vi "Main VI.vi"(0 "Available Test":string(tree), 1 "Status and graph":bool, 5 "Home":bool, 7 "Mode selection":bool, 9 "Configuration":bool, 11 "Error In":errorcluster, 12 "Run Test":bool) -> (4 "Status":string, 15 "Error Out":errorcluster)   [LabVIEW 2020, in "ADC DAC Test Measurement.lvlib"]
doc: "Main interface VI to perform the tests. It performs INL and DNL Test. It contains individual button to load its corresponding page."
uses:
  ADC DAC Test Measurement.lvlib
  Typedef/Queue Operation.ctl
  Typedef/Data Line.ctl
  Class/Test/Parent/Test.lvclass
  Typedef/User event controls.ctl
  <vilib>/Utility/config.llb/Read Key (Boolean).vi
  <vilib>/Utility/config.llb/NI_LVConfig.lvlib
panel:
  out "Graph Pic":picture
  out "Config Pic":picture
  out "Mode Pic":picture
  out "Home Pic":picture
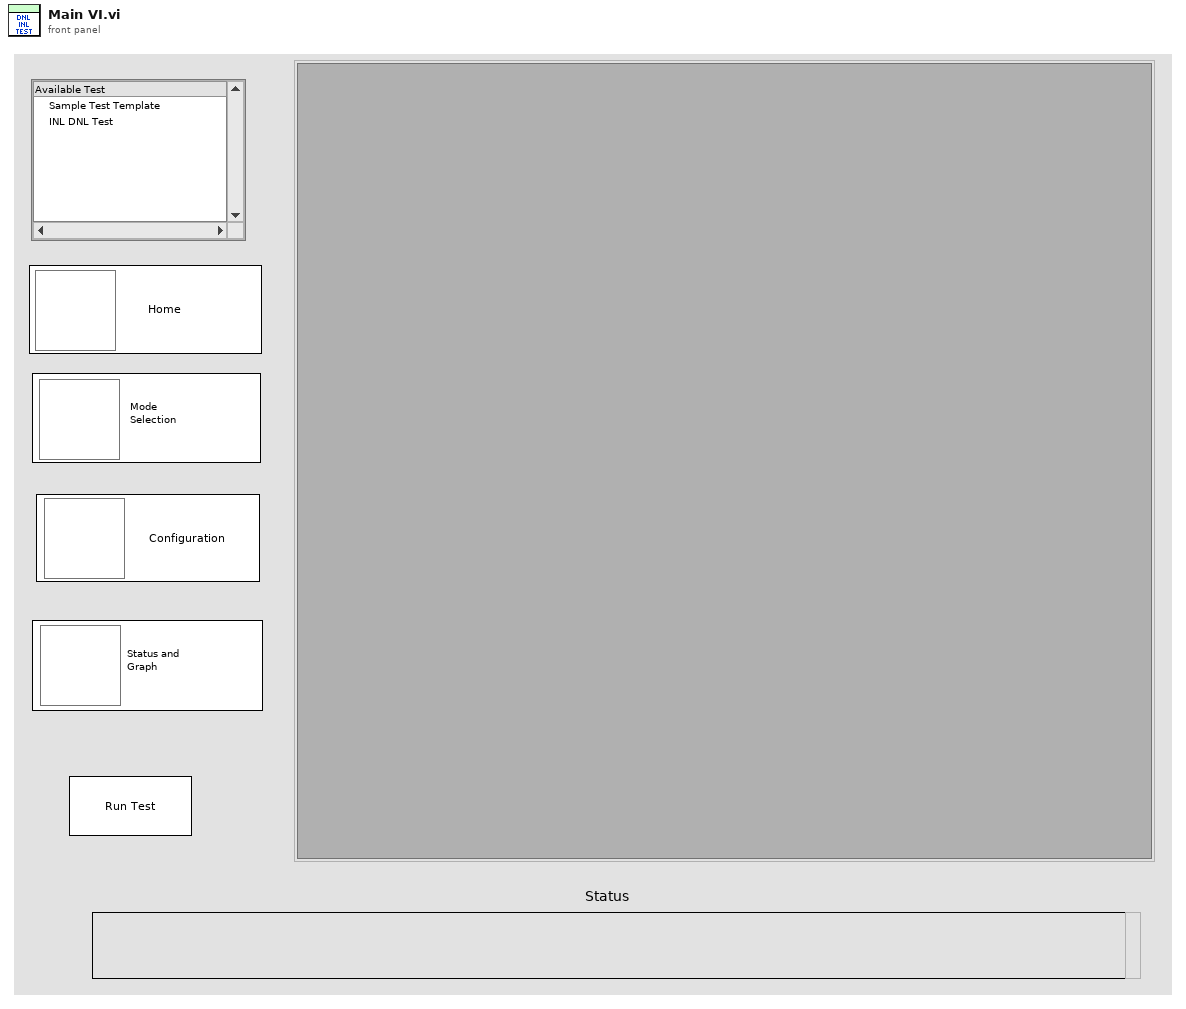
[diagram p1: front panel]
types:
  T1 = typedef "ADC DAC Test Measurement.lvlib/Data Line.ctl" = cluster{"DVR":refnum<data-value>, "Subpanel Ref":refnum<vi>, "Class Selected?":bool, "Status Msg":string, "Test Name":string, "Debug Status":bool}
  T2 = typedef "ADC DAC Test Measurement.lvlib/Queue Operation.ctl" = enum16{"Create Queue", "Enqueue", "Dequeue", "Enstack", "Flush Queue", "Release Queue"}
  T3 = typedef "ADC DAC Test Measurement.lvlib/User event controls.ctl" = enum16{"Create", "Generate", "Run Test", "Get Ref", "Destroy"}
  T4 = typedef "NI_LVConfig.lvlib/Config Data RefNum.ctl" = refnum<k1>
  T5 = typedef "imagedata.ctl" = cluster{"image type":i32, "image depth":i32, "image":u8[], "mask":u8[], "colors":u32[], "Rectangle":cluster{"left":i16, "top":i16, "right":i16, "bottom":i16}}
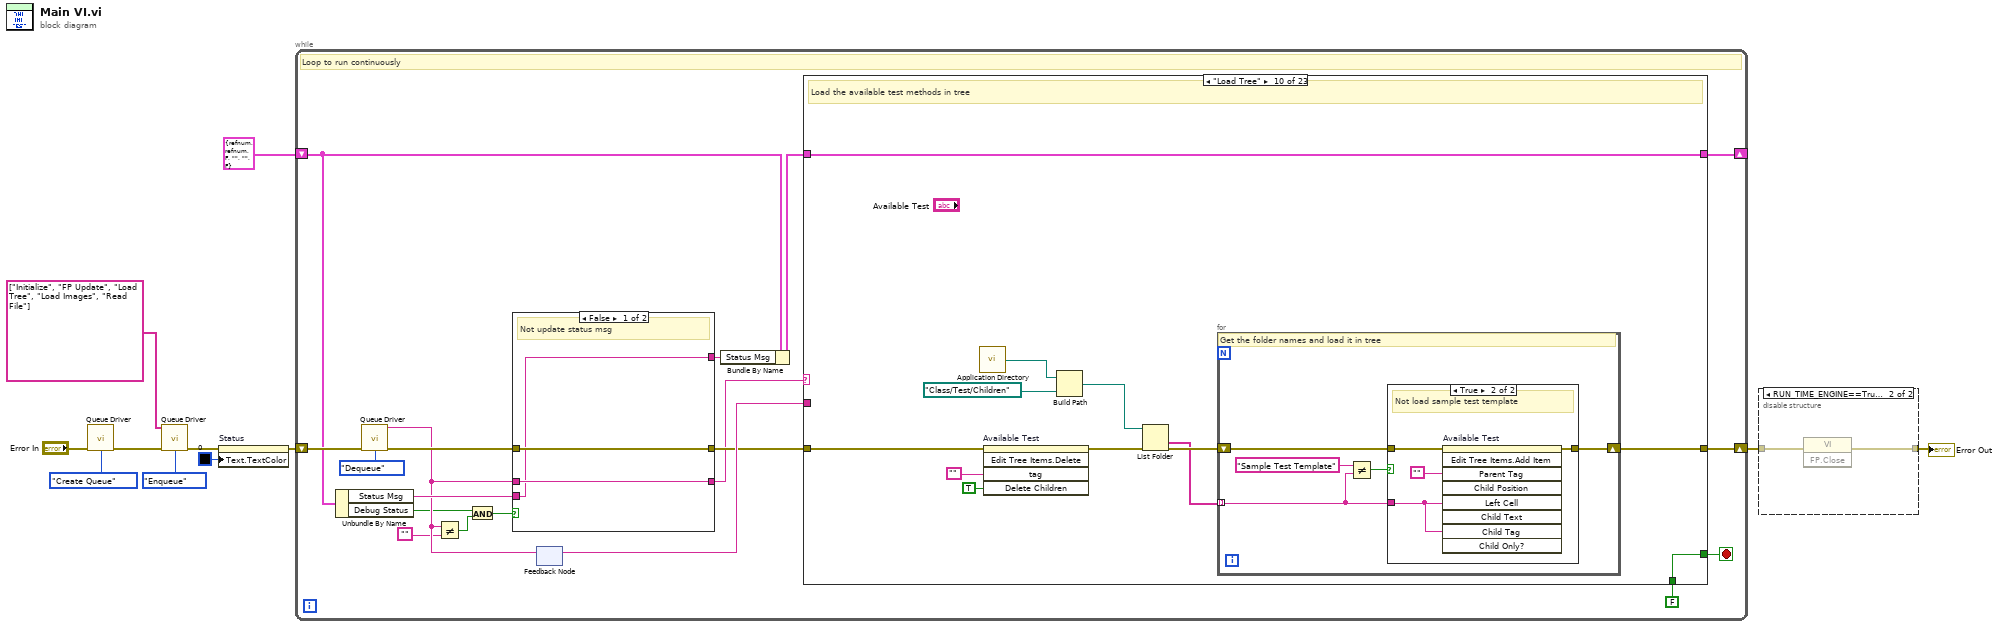
[diagram p0: block diagram]
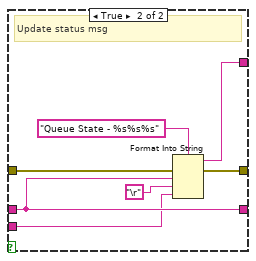
[diagram p3: hidden frame]
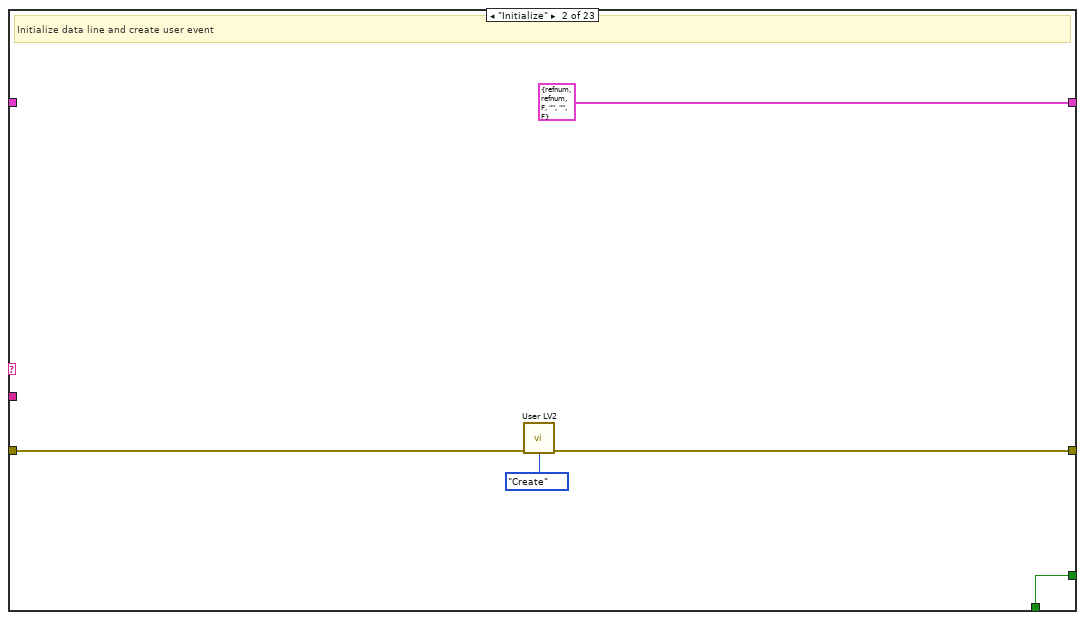
[diagram p5: hidden frame]
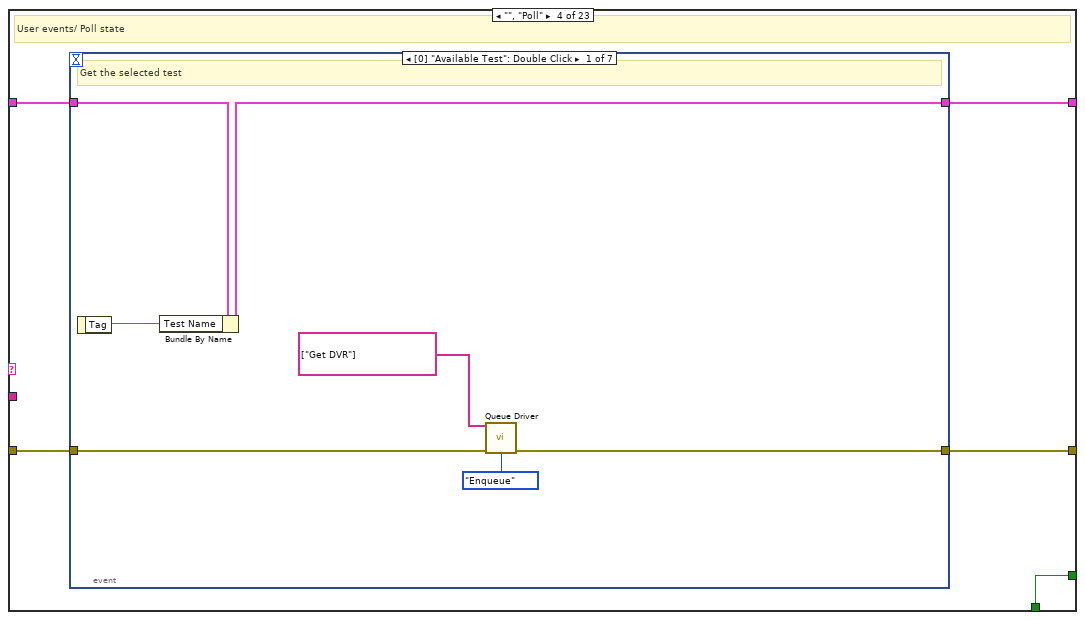
[diagram p7: hidden frame]
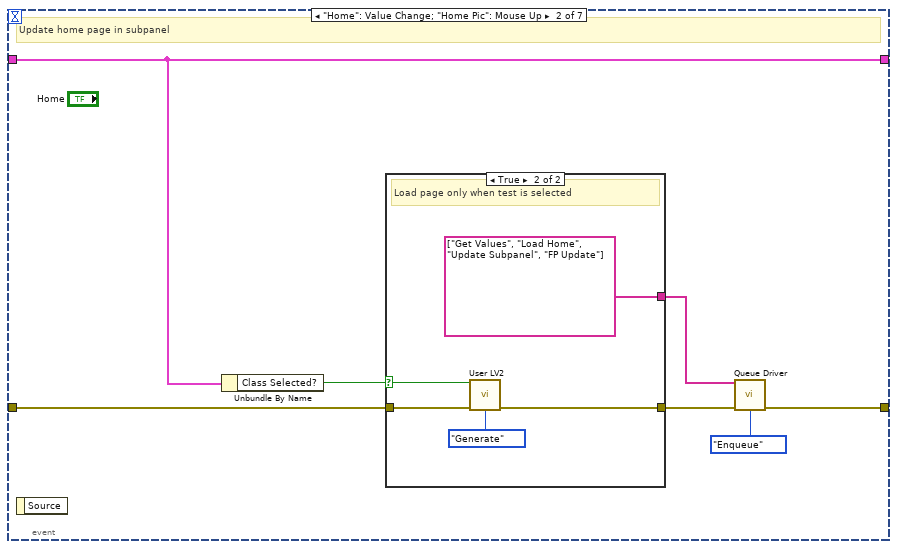
[diagram p8: hidden frame]
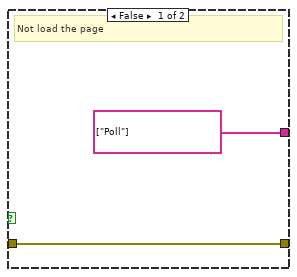
[diagram p9: hidden frame]
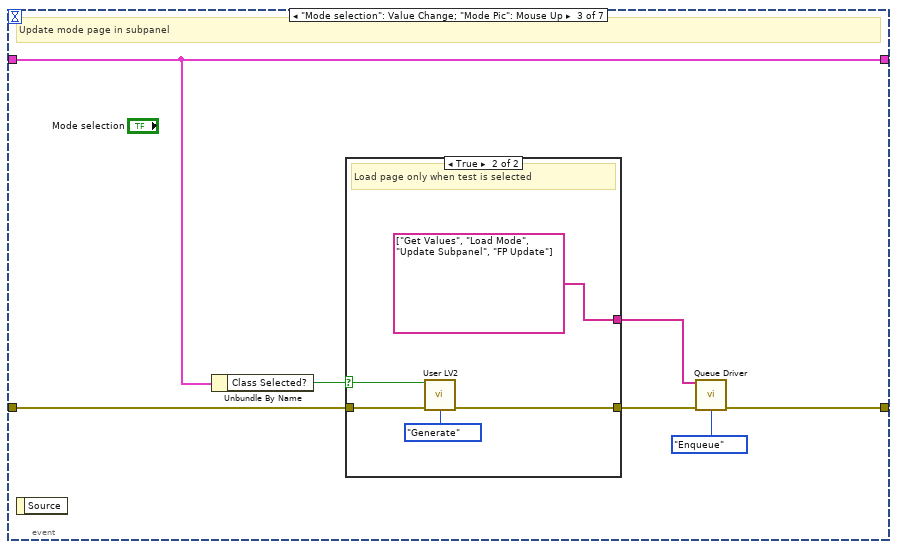
[diagram p10: hidden frame]
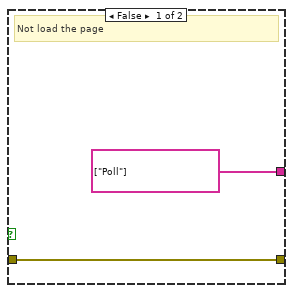
[diagram p11: hidden frame]
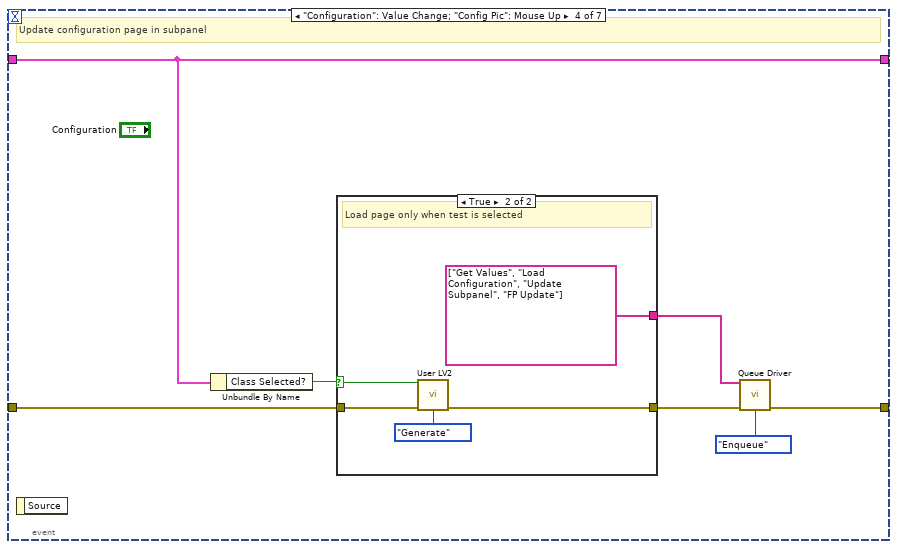
[diagram p12: hidden frame]
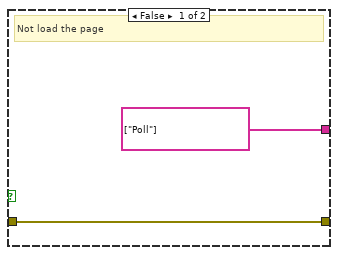
[diagram p13: hidden frame]
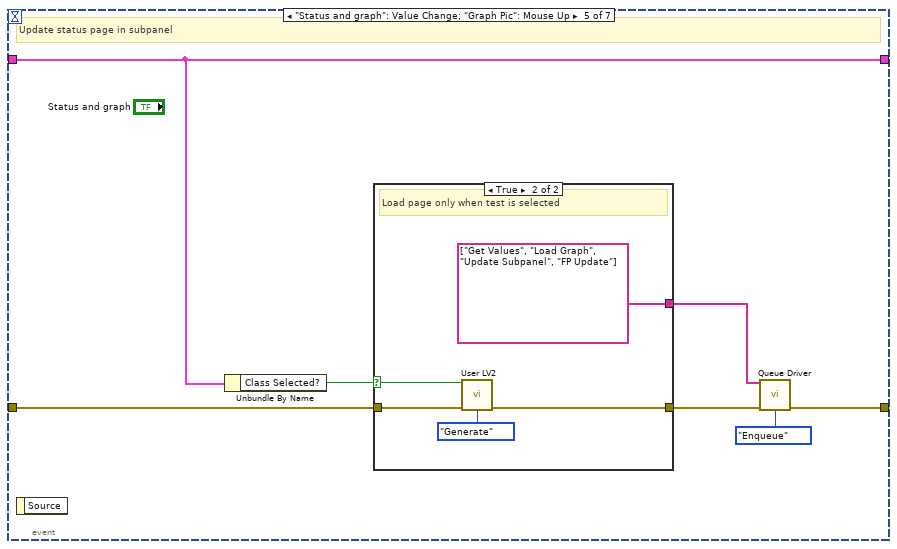
[diagram p14: hidden frame]
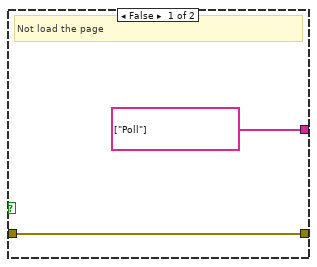
[diagram p15: hidden frame]
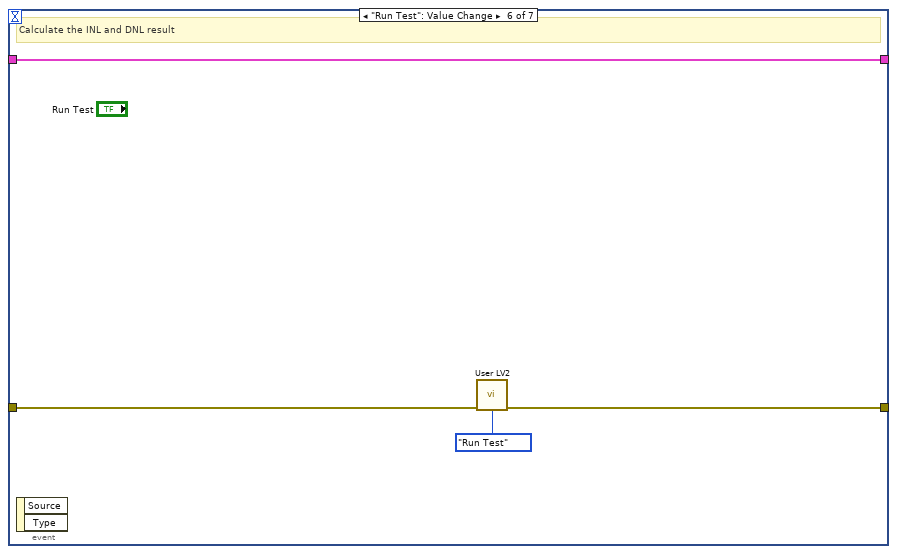
[diagram p16: hidden frame]
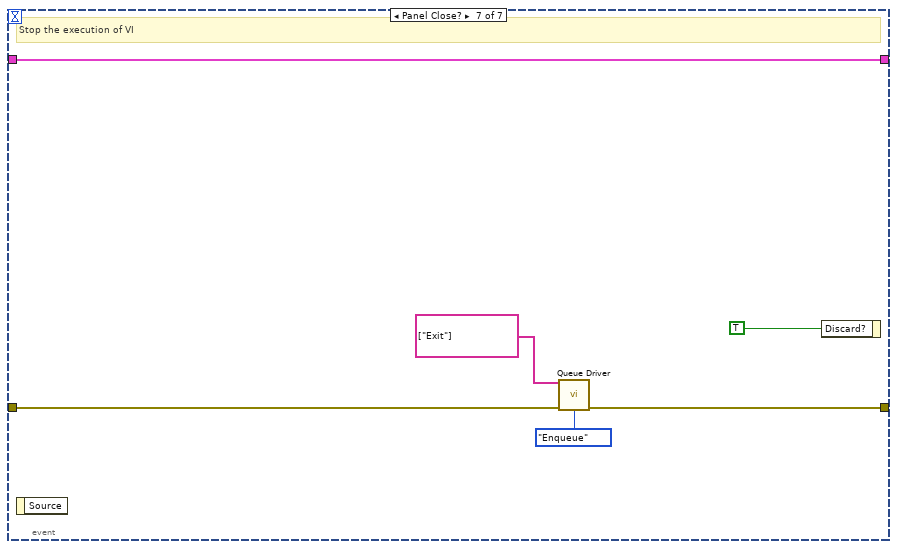
[diagram p17: hidden frame]
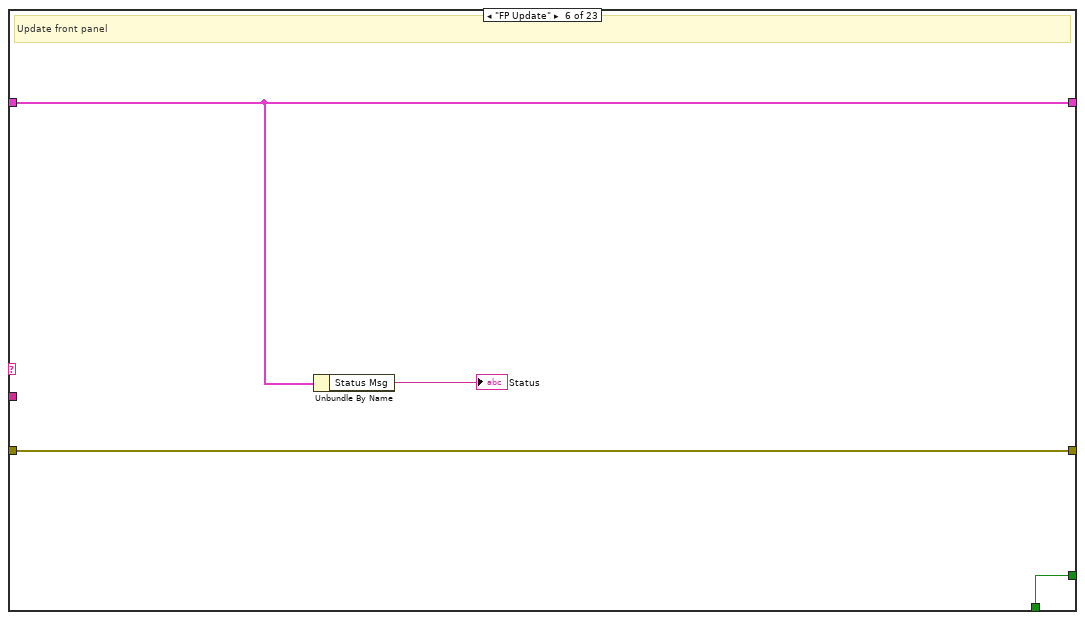
[diagram p19: hidden frame]
diagram:
  n1 = call "Queue Driver.vi"("Error In"="Error In", "Queue Operation"=Queue_Operation."Create Queue") -> ("Error Out"=w9:errorcluster)  [unwired: 12 in, 1 out]
  n2 = call "Queue Driver.vi"("States"=string[] ["Initialize", "FP Update", "Load Tree", "Load Images", "Read File"], "Error In"=w9, "Queue Operation"=Queue_Operation."Enqueue") -> ("Error Out"=w6:errorcluster)  [unwired: 11 in, 1 out]
  n3 = property on="Status" class="Str"(error in=w6, "Text.TextColor"=u32 0 ("Text.Text Colors:Text Color")) -> (error out=w4:errorcluster)  [unwired: 1 in, 1 out]
  n4 = while {
    shift-right: [w27] -> w2
    shift-left: w4 -> [w30]
    shift-right: [w24] -> _
    shift-left: T1 {"DVR"=refnum, "Subpanel Ref"=refnum, "Class Selected?"=FALSE, "Status Msg"="", "Test Name"="", "Debug Status"=FALSE} ("Data Line") -> [w19]
    stop <- w25 stop-if-true
    # "Loop to run continuously"
    n5 = Unbundle By Name(w19) -> ("Status Msg"=w20:string, "Debug Status"=w14:bool)
    n6 = call "Queue Driver.vi"("Error In"=w30, "Queue Operation"=Queue_Operation."Dequeue") -> ("Dequeue Element"=w16:string, "Error Out"=w23:errorcluster)  [unwired: 12 in]
    n7 = Not Equal?(x=w16, y="") -> (x != y?=w13:bool)
    n8 = And(x=w14, y=w13) -> (x .and. y?=w12:bool)
    n9 = case shown="False" w12 {
      tunnel: w16 -> [w32 w37]
      tunnel: [w33 w39] -> w22
      tunnel: w23 -> [w33 w40]
      tunnel: [w32 w37] -> w21
      tunnel: w20 -> [w31 w35]
      tunnel: [w31 w34] -> w18
      frame False {
        # "Not update status msg"
      }
      frame True {
        # "Update status msg"
        n10 = Format Into String(format string="Queue State - %s%s%s", error in=w40, w37, "\r", w35) -> (resulting string=w34:string, error out=w39:errorcluster)  [unwired: 1 in]
      }
    }
    n11 = feedback-in #1(w16) -> ()
    n12 = feedback #1() -> (w28:string)  [unwired: 1 in]
    n13 = Bundle By Name(cluster=w19, "Status Msg"=w18) -> (w17:T1)
    n14 = case shown="\"Load Tree\"" w21 {
      selector: w21 -> [_ _ _ _ _ _ _ _ _ _ _ _ _ _ _ _ _ _ _ _ _ _ w347]
      tunnel: w28 -> [_ _ _ _ _ _ _ _ _ _ _ _ _ _ _ _ _ _ w306 _ _ _ _]
      tunnel: w22 -> [w43 w48 w51 w56 w132 w133 w139 w150 w165 w201 w236 w237 w251 w258 w267 w272 w278 w284 w309 w312 w329 w336 w350]
      tunnel: [w43 w46 w51 w55 w132 w133 w139 w140 w155 w199 w236 w243 w245 w257 w262 w269 w274 w284 w285 w312 w325 w336 w338] -> w27
      tunnel: FALSE -> [w42 w47 w50 w54 w131 w136 w138 w154 w166 w206 w235 w244 w252 w260 w268 w273 w281 w283 w293 w311 _ w335 w351]
      tunnel: [w42 w47 w50 w54 w131 w136 w138 w154 w166 w206 w235 w244 w252 w260 w268 w273 w281 w283 w293 w311 TRUE ("T button?") w335 w351] -> w25
      tunnel: w17 -> [w41 _ w49 w53 w130 w135 w137 w143 w160 w205 w234 w241 w249 w256 w265 w271 w280 w282 w289 w310 w318 w334 w337]
      tunnel: [w41 T1 {"DVR"=refnum, "Subpanel Ref"=refnum, "Class Selected?"=FALSE, "Status Msg"="", "Test Name"="", "Debug Status"=FALSE} ("Data Line") w49 w52 w130 w135 w137 w141 w159 w205 w234 w238 w247 w253 w261 w271 w279 w282 w287 w310 w318 w334 w337] -> w24
      frame "/****Initialize****/" {
        # "Splitter"
      }
      frame "Initialize" {
        # "Initialize data line and create user event"
        n15 = call "User LV2.vi"("Error In"=w48, "User event controls"=User_event_controls."Create") -> ("Error Out"=w46:errorcluster)  [unwired: 11 in, 2 out]
      }
      frame "/****User inputs****/" {
        # "Splitter"
      }
      frame "", "Poll" {
        # "User events/ Poll state"
        n16 = event shown="[0] \"Available Test\": Double Click" {
          selector: _ -> [_ _ _ _ _ _ _]
          dyn-events: _ -> [_ _ _ _ _ _ _]
          timeout: _ -> [_ _ _ _ _ _ _]
          tunnel: w56 -> [w60 w67 w81 w95 w109 w123 w127]
          tunnel: [w59 w70 w82 w96 w110 w121 w126] -> w55
          tunnel: w53 -> [w63 w65 w79 w93 w107 w122 w129]
          tunnel: [w62 w65 w79 w93 w107 w122 w129] -> w52
          event "Available Test": Double Click {
            # "Get the selected test"
            n17 = event-data() -> ("Tag"=w61:string)  [unwired: 1 in]
            n18 = Bundle By Name(cluster=w63, "Test Name"=w61) -> (w62:T1)
            n19 = call "Queue Driver.vi"("States"=string[] ["Get DVR"], "Error In"=w60, "Queue Operation"=Queue_Operation."Enqueue") -> ("Error Out"=w59:errorcluster)  [unwired: 11 in, 1 out]
          }
          event "Home": Value Change; "Home Pic": Mouse Up {
            # "Update home page in subpanel"
            n20 = event-data() -> ()  [unwired: 1 in, 1 out]
            n21 = Unbundle By Name(w65) -> ("Class Selected?"=w64:bool)
            n22 = case shown="True" w64 {
              selector: w64 -> [_ w73]
              tunnel: [string[] ["Poll"] ("States") string[] ["Get Values", "Load Home", "Update Subpanel", "FP Update"] ("States")] -> w68
              tunnel: w67 -> [w71 w76]
              tunnel: [w71 w75] -> w66
              frame False {
                # "Not load the page"
              }
              frame True {
                # "Load page only when test is selected"
                n23 = call "User LV2.vi"("Stop"=w73, "Error In"=w76, "User event controls"=User_event_controls."Generate") -> ("Error Out"=w75:errorcluster)  [unwired: 10 in, 2 out]
              }
            }
            n24 = call "Queue Driver.vi"("States"=w68, "Error In"=w66, "Queue Operation"=Queue_Operation."Enqueue") -> ("Error Out"=w70:errorcluster)  [unwired: 11 in, 1 out]
          }
          event "Mode selection": Value Change; "Mode Pic": Mouse Up {
            # "Update mode page in subpanel"
            n25 = event-data() -> ()  [unwired: 1 in, 1 out]
            n26 = Unbundle By Name(w79) -> ("Class Selected?"=w78:bool)
            n27 = case shown="True" w78 {
              selector: w78 -> [_ w87]
              tunnel: [string[] ["Poll"] ("States") string[] ["Get Values", "Load Mode", "Update Subpanel", "FP Update"] ("States")] -> w83
              tunnel: [w85 w89] -> w80
              tunnel: w81 -> [w85 w91]
              frame False {
                # "Not load the page"
              }
              frame True {
                # "Load page only when test is selected"
                n28 = call "User LV2.vi"("Stop"=w87, "Error In"=w91, "User event controls"=User_event_controls."Generate") -> ("Error Out"=w89:errorcluster)  [unwired: 10 in, 2 out]
              }
            }
            n29 = call "Queue Driver.vi"("States"=w83, "Error In"=w80, "Queue Operation"=Queue_Operation."Enqueue") -> ("Error Out"=w82:errorcluster)  [unwired: 11 in, 1 out]
          }
          event "Configuration": Value Change; "Config Pic": Mouse Up {
            # "Update configuration page in subpanel"
            n30 = event-data() -> ()  [unwired: 1 in, 1 out]
            n31 = Unbundle By Name(w93) -> ("Class Selected?"=w92:bool)
            n32 = case shown="True" w92 {
              selector: w92 -> [_ w101]
              tunnel: [string[] ["Poll"] ("States") string[] ["Get Values", "Load Configuration", "Update Subpanel", "FP Update"] ("States")] -> w97
              tunnel: w95 -> [w99 w105]
              tunnel: [w99 w103] -> w94
              frame False {
                # "Not load the page"
              }
              frame True {
                # "Load page only when test is selected"
                n33 = call "User LV2.vi"("Stop"=w101, "Error In"=w105, "User event controls"=User_event_controls."Generate") -> ("Error Out"=w103:errorcluster)  [unwired: 10 in, 2 out]
              }
            }
            n34 = call "Queue Driver.vi"("States"=w97, "Error In"=w94, "Queue Operation"=Queue_Operation."Enqueue") -> ("Error Out"=w96:errorcluster)  [unwired: 11 in, 1 out]
          }
          event "Status and graph": Value Change; "Graph Pic": Mouse Up {
            # "Update status page in subpanel"
            n35 = event-data() -> ()  [unwired: 1 in, 1 out]
            n36 = Unbundle By Name(w107) -> ("Class Selected?"=w106:bool)
            n37 = case shown="True" w106 {
              selector: w106 -> [_ w115]
              tunnel: [string[] ["Poll"] ("States") string[] ["Get Values", "Load Graph", "Update Subpanel", "FP Update"] ("States")] -> w111
              tunnel: [w113 w117] -> w108
              tunnel: w109 -> [w113 w119]
              frame False {
                # "Not load the page"
              }
              frame True {
                # "Load page only when test is selected"
                n38 = call "User LV2.vi"("Stop"=w115, "Error In"=w119, "User event controls"=User_event_controls."Generate") -> ("Error Out"=w117:errorcluster)  [unwired: 10 in, 2 out]
              }
            }
            n39 = call "Queue Driver.vi"("States"=w111, "Error In"=w108, "Queue Operation"=Queue_Operation."Enqueue") -> ("Error Out"=w110:errorcluster)  [unwired: 11 in, 1 out]
          }
          event "Run Test": Value Change {
            # "Calculate the INL and DNL result"
            n40 = event-data() -> ()  [unwired: 1 in, 2 out]
            n41 = call "User LV2.vi"("Error In"=w123, "User event controls"=User_event_controls."Run Test") -> ("Error Out"=w121:errorcluster)  [unwired: 11 in, 2 out]
          }
          event Panel Close? {
            # "Stop the execution of VI"
            n42 = event-data() -> ()  [unwired: 1 in, 1 out]
            n43 = call "Queue Driver.vi"("States"=string[] ["Exit"], "Error In"=w127, "Queue Operation"=Queue_Operation."Enqueue") -> ("Error Out"=w126:errorcluster)  [unwired: 11 in, 1 out]
            n44 = event-data("Discard?"=TRUE) -> ()  [unwired: 1 in, 1 out]
          }
        }
      }
      frame "/****Front panel updates****/" {
        # "Splitter"
      }
      frame "FP Update" {
        # "Update front panel"
        n45 = Unbundle By Name(w135) -> ("Status Msg"=→"Status":string)
      }
      frame "/****Functionality****/" {
        # "Splitter"
      }
      frame "Read File" {
        # "Read ini file for status message update"
        n46 = call <vilib>:"Application Directory.vi"() -> ("Application Directory"=w153:path)
        n47 = Build Path(base path=w153, name or relative path=path "Debug File/Debug Mode.ini") -> (appended path=w151:path)
        n48 = call <vilib>:"Open Config Data.vi"("error in (no error)"=w150, "configuration file path"=w151) -> ("error out"=w149:errorcluster, "refnum"=w148:T4)  [unwired: 7 in, 1 out]
        n49 = call-poly <vilib>:"Read Key.vi"("section"="Debug", "error in (no error)"=w149, "key"="Status", "refnum"=w148) -> ("error out"=w145:errorcluster, "value"=w142:bool, "refnum out"=w144:T4)  [unwired: 4 in, 1 out]
        n50 = Bundle By Name(cluster=w143, "Debug Status"=w142) -> (w141:T1)
        n51 = call <vilib>:"Close Config Data.vi"("error in (no error)"=w145, "refnum"=w144) -> ("error out"=w140:errorcluster)  [unwired: 8 in, 1 out]
      }
      frame "Get DVR" {
        # "Generate DVR for selected test method"
        n52 = Unbundle By Name(w160) -> ("DVR"=w164:refnum<data-value>, "Test Name"=w163:string)
        n53 = Empty String/Path?(string/path=w163) -> (empty?=w162:bool)
        n54 = case shown="False" w162 {
          selector: w162 -> [w171 w187]
          tunnel: w165 -> [w179 w190]
          tunnel: [w169 w186] -> w156
          tunnel: w163 -> [w173 _]
          tunnel: [w174 refnum<data-value> refnum ("DVR Out")] -> w158
          tunnel: w164 -> [_ w181]
          tunnel: [w171 w187] -> w157
          frame False {
            # "When the tag is not empty create DVR for the test"
            n55 = Format Into String(format string="Class\\\\Test\\\\Children\\\\%s\\\\%s.lvclass", error in=w179, w173, w173) -> (resulting string=w176:string, error out=w175:errorcluster)  [unwired: 1 in]
            n56 = call <vilib>:"Application Directory.vi"() -> ("Application Directory"=w177:path)
            n57 = Build Path(base path=w177, name or relative path=w176) -> (appended path=w172:path)
            n58 = call "Get DVR for Path.vi"("Error in"=w175, "Class path"=w172) -> ("Error out"=w170:errorcluster, "DVR Out"=w174:refnum<data-value>)  [unwired: 8 in]
            n59 = call "Queue Driver.vi"("States"=string[] ["Load Home", "Update Subpanel", "FP Update"], "Error In"=w170, "Queue Operation"=Queue_Operation."Enqueue") -> ("Error Out"=w169:errorcluster)  [unwired: 11 in, 1 out]
          }
          frame True {
            # "When the tag is empty remove the VI"
            n60 = Not A Number/Path/Refnum?(number/path/refnum=w181) -> (NaN/Path/Refnum?=w182:bool)
            n61 = case shown="False" w182 {
              tunnel: w190 -> [w193 w194]
              tunnel: [w192 w194] -> w183
              tunnel: w181 -> [w191 _]
              frame False {
                n62 = Delete Data Value Reference(data value reference=w191, error in=w193) -> (error out=w192:errorcluster)  [unwired: 1 out]
              }
              frame True {
              }
            }
            n63 = call "User LV2.vi"("Stop"=w187, "Error In"=w183, "User event controls"=User_event_controls."Generate") -> ("Error Out"=w189:errorcluster)  [unwired: 10 in, 2 out]
            n64 = call "Queue Driver.vi"("States"=string[] ["FP Update"], "Error In"=w189, "Queue Operation"=Queue_Operation."Enqueue") -> ("Error Out"=w186:errorcluster)  [unwired: 11 in, 1 out]
          }
        }
        n65 = Not(x=w157) -> (.not. x?=w161:bool)
        n66 = invoke on="Sub Panel" class="SubPnl" method="Remove VI"(error in=w156) -> (error out=w155:errorcluster)  [unwired: 2 in, 2 out]
        n67 = Bundle By Name(cluster=w160, "DVR"=w158, "Class Selected?"=w161) -> (w159:T1)
      }
      frame "Load Tree" {
        # "Load the available test methods in tree"
        n68 = call <vilib>:"Application Directory.vi"() -> ("Application Directory"=w204:path)
        n69 = invoke on="Available Test" class="Tree (strict)" method="Edit Tree Items.Delete"(error in=w201, "tag"="", "Delete Children"=TRUE ("Delete Children?")) -> (error out=w197:errorcluster)  [unwired: 2 in, 4 out]
        n70 = Build Path(base path=w204, name or relative path=path "Class/Test/Children") -> (appended path=w202:path)
        n71 = List Folder(path=w202, error in=w197) -> (folder names=w198:string[], error out=w200:errorcluster)  [unwired: 2 in, 2 out]
        n72 = for {
          shift-right: [w210] -> w199
          shift-left: w200 -> [w211]
          tunnel: w198 -> [w208] mode=indexing
          # "Get the folder names and load it in tree"
          n73 = Not Equal?(x="Sample Test Template", y=w208) -> (x != y?=w209:bool)
          n74 = case shown="True" w209 {
            tunnel: w211 -> [w212 w216]
            tunnel: [w212 w215] -> w210
            tunnel: w208 -> [_ w213]
            frame False {
            }
            frame True {
              # "Not load sample test template"
              n75 = invoke on="Available Test" class="Tree (strict)" method="Edit Tree Items.Add Item"(error in=w216, "Parent Tag"="", "Left Cell"=w213, "Child Tag"=w213) -> (error out=w215:errorcluster)  [unwired: 5 in, 8 out]
            }
          }
        }
      }
      frame "Load Images" {
        # "Load images to the buttons"
        n76 = call <vilib>:"Application Directory.vi"() -> ("Application Directory"=w217:path)
        n77 = Build Path(base path=w217, name or relative path=path "Images/Home.png") -> (appended path=w231:path)
        n78 = Build Path(base path=w217, name or relative path=path "Images/Mode Selection.png") -> (appended path=w230:path)
        n79 = Build Path(base path=w217, name or relative path=path "Images/Configuration.png") -> (appended path=w224:path)
        n80 = Build Path(base path=w217, name or relative path=path "Images/Status and Graph.png") -> (appended path=w221:path)
        n81 = call <vilib>:"Read PNG File.vi"("path to PNG file"=w231) -> ("image data"=w233:T5)  [unwired: 8 in, 2 out]
        n82 = call <vilib>:"Read PNG File.vi"("path to PNG file"=w230) -> ("image data"=w229:T5)  [unwired: 8 in, 2 out]
        n83 = call <vilib>:"Read PNG File.vi"("path to PNG file"=w224) -> ("image data"=w225:T5)  [unwired: 8 in, 2 out]
        n84 = call <vilib>:"Read PNG File.vi"("path to PNG file"=w221) -> ("image data"=w222:T5)  [unwired: 8 in, 2 out]
        n85 = call <vilib>:"Draw Flattened Pixmap.vi"("image data"=w233) -> ("new picture"=→"Home Pic":picture)  [unwired: 8 in]
        n86 = call <vilib>:"Draw Flattened Pixmap.vi"("image data"=w229) -> ("new picture"=→"Mode Pic":picture)  [unwired: 8 in]
        n87 = call <vilib>:"Draw Flattened Pixmap.vi"("image data"=w225) -> ("new picture"=→"Config Pic":picture)  [unwired: 8 in]
        n88 = call <vilib>:"Draw Flattened Pixmap.vi"("image data"=w222) -> ("new picture"=→"Graph Pic":picture)  [unwired: 8 in]
      }
      frame "Load Home" {
        # "Load hoem page"
        n89 = Unbundle By Name(w241) -> ("DVR"=w242:refnum<data-value>)
        n90 = call "Home_Ref_API.vi"("DVR In"=w242, "Error In"=w237) -> ("DVR Out"=w240:refnum<data-value>, "VI Ref"=w239:refnum<vi>, "Error Out"=w243:errorcluster)  [unwired: 11 in]
        n91 = Bundle By Name(cluster=w241, "DVR"=w240, "Subpanel Ref"=w239) -> (w238:T1)
      }
      frame "Load Mode" {
        # "Load mode page"
        n92 = Unbundle By Name(w249) -> ("DVR"=w250:refnum<data-value>)
        n93 = call "Mode_Ref_API.vi"("DVR In"=w250, "Error In"=w251) -> ("DVR Out"=w248:refnum<data-value>, "VI Ref"=w246:refnum<vi>, "Error out"=w245:errorcluster)  [unwired: 11 in]
        n94 = Bundle By Name(cluster=w249, "DVR"=w248, "Subpanel Ref"=w246) -> (w247:T1)
      }
      frame "Load Configuration" {
        # "Load configuration page"
        n95 = Unbundle By Name(w256) -> ("DVR"=w259:refnum<data-value>)
        n96 = call "Configuration_Ref_API.vi"("DVR In"=w259, "Error In"=w258) -> ("DVR Out"=w255:refnum<data-value>, "VI Ref"=w254:refnum<vi>, "Error Out"=w257:errorcluster)  [unwired: 11 in]
        n97 = Bundle By Name(cluster=w256, "DVR"=w255, "Subpanel Ref"=w254) -> (w253:T1)
      }
      frame "Load Graph" {
        # "Load graph page"
        n98 = Unbundle By Name(w265) -> ("DVR"=w266:refnum<data-value>)
        n99 = call "Status_Ref_API.vi"("DVR In"=w266, "Error In"=w267) -> ("DVR Out"=w264:refnum<data-value>, "VI Ref"=w263:refnum<vi>, "Error Out"=w262:errorcluster)  [unwired: 11 in]
        n100 = Bundle By Name(cluster=w265, "DVR"=w264, "Subpanel Ref"=w263) -> (w261:T1)
      }
      frame "Update Subpanel" {
        # "Load VI reference into subpanel"
        n101 = Unbundle By Name(w271) -> ("Subpanel Ref"=w270:refnum<vi>)
        n102 = invoke on="Sub Panel" class="SubPnl" method="Insert VI"(error in=w272, "VI Ref"=w270) -> (error out=w269:errorcluster)  [unwired: 2 in, 3 out]
      }
      frame "Get Values" {
        # "Get the values from the previous loaded page and update values in currently loaded page"
        n103 = Unbundle By Name(w280) -> ("DVR"=w277:refnum<data-value>, "Subpanel Ref"=w275:refnum<vi>)
        n104 = call "Get_Reference_API.vi"("DVR"=w277, "Subpanel Ref"=w275, "Error In"=w278) -> ("DVR Out"=w276:refnum<data-value>, "Error Out"=w274:errorcluster)  [unwired: 11 in]
        n105 = Bundle By Name(cluster=w280, "DVR"=w276) -> (w279:T1)
      }
      frame "/****Error****/" {
        # "Splitter"
      }
      frame "Error" {
        # "Error occurs"
        n106 = Unbundle By Name(w309) -> ("code"=w305:i32, "source"=w304:string)
        n107 = call <vilib>:"Clear Errors.vi"("error in (no error)"=w309, "specific error code to clear (0: all)"=w305) -> ("error out"=w308:errorcluster)  [unwired: 4 in, 1 out]
        n108 = Format Into String(format string="Error Occurred in \"%s\" State \n\nError Code: %d\nDescription: %s\n\nDo you want to stop or continue? \n", error in=w308, w306, w305, w304) -> (resulting string=w303:string, error out=w297:errorcluster)  [unwired: 1 in]
        n109 = Two Button Dialog(message=w303, 1:"Continue" ("F button name (\"Cancel\")"), 2:"Stop" ("T button name (\"OK\")")) -> (T button?=w300:bool)
        n110 = property on="Status" class="Str"("Text.TextColor"=u32 16711680 ("Text.Text Colors:Text Color")) -> ()  [unwired: 2 in, 2 out]
        n111 = Select(t=string[] ["Exit", "FP Update"] ("States"), s=w300, f=string[] ["FP Update"] ("States")) -> (s? t:f=w294:string[])
        n112 = Unbundle By Name(w289) -> ("Status Msg"=w290:string)
        n113 = call "Queue Driver.vi"("States"=w294, "Error In"=w297, "Queue Operation"=Queue_Operation."Enstack") -> ("Error Out"=w296:errorcluster)  [unwired: 11 in, 1 out]
        n114 = Format Into String(format string="\"ERROR OCCURRED\" %s%s", error in=w296, "\r", w290) -> (resulting string=w288:string, error out=w285:errorcluster)  [unwired: 1 in]
        n115 = Bundle By Name(cluster=w289, "Status Msg"=w288) -> (w287:T1)
      }
      frame "/****Exit****/" {
        # "Splitter"
      }
      frame "Exit" {
        # "Delete reference if it is not\na empty reference line"
        # "Stop the execution of VI"
        n116 = Unbundle By Name(w318) -> ("DVR"=w317:refnum<data-value>, "Subpanel Ref"=w313:refnum<vi>)
        n117 = call "User LV2.vi"("Stop"=TRUE, "Error In"=w329, "User event controls"=User_event_controls."Generate") -> ("Error Out"=w322:errorcluster)  [unwired: 10 in, 2 out]
        n118 = call "User LV2.vi"("Error In"=w322, "User event controls"=User_event_controls."Destroy") -> ("Error Out"=w316:errorcluster)  [unwired: 11 in, 2 out]
        n119 = Not A Number/Path/Refnum?(number/path/refnum=w313) -> (NaN/Path/Refnum?=w314:bool)
        n120 = case shown="False" w314 {
          tunnel: w316 -> [w332 w333]
          tunnel: [w331 w333] -> w315
          tunnel: w313 -> [w330 _]
          frame False {
            n121 = Close Reference(reference=w330, error in (no error)=w332) -> (error out=w331:errorcluster)
          }
          frame True {
          }
        }
        n122 = call "Delete DVR.vi"("Error in"=w315, "DVR In"=w317) -> ("error out"=w319:errorcluster)  [unwired: 9 in]
        n123 = call "Queue Driver.vi"("Error In"=w319, "Queue Operation"=Queue_Operation."Flush Queue") -> ("Error Out"=w327:errorcluster)  [unwired: 12 in, 1 out]
        n124 = call "Queue Driver.vi"("Error In"=w327, "Queue Operation"=Queue_Operation."Release Queue") -> ("Error Out"=w325:errorcluster)  [unwired: 12 in, 1 out]
      }
      frame "/****Developer error****/" {
        # "Splitter"
      }
      frame Default {
        # "Default state"
        n125 = Format Into String(format string="State name: %s\n\nState name not found\n\nDo you want to stop or continue?\n", error in=w350, w347) -> (resulting string=w346:string, error out=w349:errorcluster)  [unwired: 1 in]
        n126 = Two Button Dialog(message=w346, 1:"Continue" ("F button name (\"Cancel\")"), 2:"Stop" ("T button name (\"OK\")")) -> (T button?=w343:bool)
        n127 = Select(t=string[] ["Exit"] ("States"), s=w343, f=string[] ["Poll"] ("States")) -> (s? t:f=w340:string[])
        n128 = call "Queue Driver.vi"("States"=w340, "Error In"=w349, "Queue Operation"=Queue_Operation."Enqueue") -> ("Error Out"=w338:errorcluster)  [unwired: 11 in, 1 out]
      }
    }
  }
  n129 = disable-structure shown="RUN_TIME_ENGINE==True" {
    disable-tunnel: w2 -> [w352 w354]
    disable-tunnel: [w352 w353] -> w1
    frame condition #0 (active) {
    }
    frame condition #1 {
      n130 = invoke class="VI" method="FP.Close"(error in=w354) -> (error out=w353:errorcluster)  [unwired: 2 in, 2 out]
    }
  }
  "Error Out" <- w1
